vi "MGI Create.vi"(8 "error in (no error)":errorcluster, 9 "Ignore Warnings? (F: Process Errors and Warnings)":bool, 10 "Error Log Directory \n(Not a Path: Shared Docs\\Caller Prefix)\n(\"\" Path: Turn off logging)":path=path "", 11 "Reporter Dialog.lvclass":refnum<class "MGI Error Reporter Dialog.lvclass">) -> (0 "error out":errorcluster, 2 "Error Log Directory Used":path, 3 "Already Running?":bool)   [LabVIEW 2020, in "MGI Error Reporter Dialog.lvclass"]
doc: "Starts an Error Reporter daemon using the optionally wired Error Reporter. If Error Handler is not wired, the MGI Error Reporter Dialog is used. If an Error Reporter daemon is already running from a top level VI, do nothing and output True for \"Already Running\".\nSee \"VI Tree.vi\" for more details.\nIf this VI is used on RT, the Dialog Class will be loaded on RT. This may cause linking and saving problems.\n\nAuthored by Shawn Walpole\nsupport@mooregoodideas.com\nwww.mooregoodideas.com\n\nCopyright (c) 2013, Moore Good Ideas, Inc.\n\nAll rights reserved.\n\nRedistribution and use in source and binary forms, with or without modification, are permitted provided that the following conditions are met:\n\n * Redistributions of source code must retain the above copyright notice, this list of conditions and the following disclaimer.\n * Redistributions in binary form must reproduce the above copyright notice, this list of conditions and the following disclaimer in the documentation and/or other materials provided with the distribution.\n * Neither the name of Moore Good Ideas, Inc. nor the names of its contributors may be used to endorse or promote products derived from this software without specific prior written permission.\n\nTHIS SOFTWARE IS PROVIDED BY THE COPYRIGHT HOLDERS AND CONTRIBUTORS \"AS IS\" AND ANY EXPRESS OR IMPLIED WARRANTIES, INCLUDING, BUT NOT LIMITED TO, THE IMPLIED WARRANTIES OF MERCHANTABILITY AND FITNESS FOR A PARTICULAR PURPOSE ARE DISCLAIMED. IN NO EVENT SHALL THE COPYRIGHT OWNER OR CONTRIBUTORS BE LIABLE FOR ANY DIRECT, INDIRECT, INCIDENTAL, SPECIAL, EXEMPLARY, OR CONSEQUENTIAL DAMAGES (INCLUDING, BUT NOT LIMITED TO, PROCUREMENT OF SUBSTITUTE GOODS OR SERVICES; LOSS OF USE, DATA, OR PROFITS; OR BUSINESS INTERRUPTION) HOWEVER CAUSED AND ON ANY THEORY OF LIABILITY, WHETHER IN CONTRACT, STRICT LIABILITY, OR TORT (INCLUDING NEGLIGENCE OR OTHERWISE) ARISING IN ANY WAY OUT OF THE USE OF THIS SOFTWARE, EVEN IF ADVISED OF THE POSSIBILITY OF SUCH DAMAGE."
uses:
  <userlib>/_MGI/Error Reporter/MGI Error Reporter Dialog/MGI Error Reporter Dialog.lvclass
  C:/Program Files/National Instruments/LabVIEW 2020/user.lib/_MGI/Error Reporter/MGI Error Reporter Base/MGI Error Reporter Base.lvclass
  <userlib>/_MGI/Error Reporter/MGI Error Reporter Base/MGI Error Reporter Base.lvclass
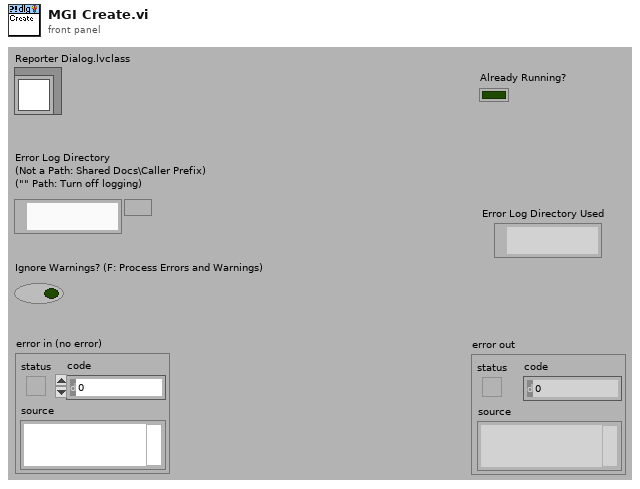
[diagram p1: front panel]
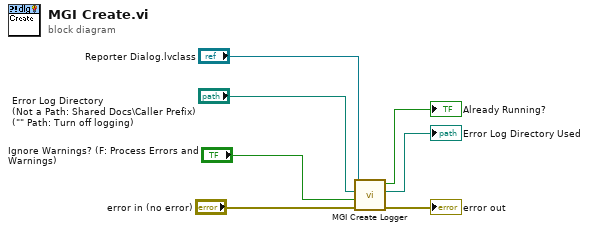
[diagram p0: block diagram]
diagram:
  n1 = call <userlib>:"MGI Create Logger.vi"("error in (no error)"="error in (no error)", "Ignore Warnings? (F: Process Errors and Warnings)"="Ignore Warnings? (F: Process Errors and Warnings)", "Error Log Directory \n(Not a Path: Shared Docs\\Caller Prefix)\n(\"\" Path: Turn off logging)"="Error Log Directory \n(Not a Path: Shared Docs\\Caller Prefix)\n(\"\" Path: Turn off logging)", "Error Reporter"="Reporter Dialog.lvclass") -> ("error out"=→"error out":errorcluster, "Error Log Directory Used"=→"Error Log Directory Used":path, "Already Running?"=→"Already Running?":bool)  [unwired: 5 out]
